vi "tableau 5 valves en liste.vi"(1 "Tableau de 5 valves":string[](array[string])=["08120001", "08120002", "08120003", "08120004", "08120005"]) -> (0 "Chaîne de 5 valves":string="08120001, 08120002, 08120003, 08120004, 08120005")   [LabVIEW 2020]
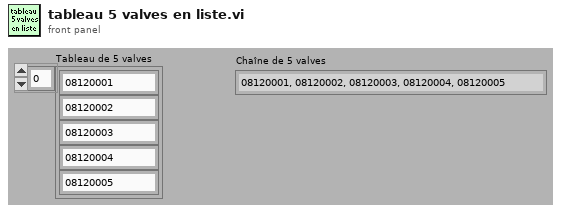
[diagram p1: front panel]
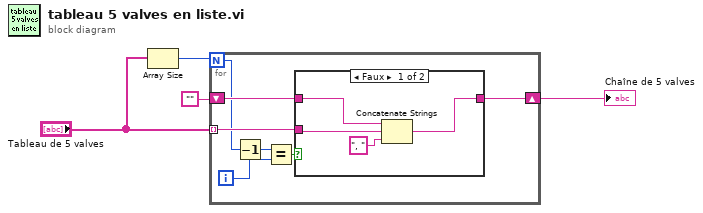
[diagram p0: block diagram]
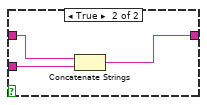
[diagram p2: hidden frame]
diagram:
  n1 = Array Size(array="Tableau de 5 valves") -> (size(s)=w3:i32)
  n2 = for {
    N: w3 -> [w7]
    tunnel: "Tableau de 5 valves" -> [w10] mode=indexing
    shift-right: [w5] -> w1
    shift-left: "" -> [w11]
    i -> [w8]
    n3 = Decrement(x=w7) -> (x-1=w6:i32)
    n4 = Equal?(x=w6, y=w8) -> (x = y?=w9:bool)
    n5 = case shown="Faux" w9 {
      tunnel: w11 -> [w14 w18]
      tunnel: w10 -> [w13 w17]
      tunnel: [w12 w16] -> w5
      frame False {
        n6 = Concatenate Strings(w14, w13, ", ") -> (w12:string)
      }
      frame True {
        n7 = Concatenate Strings(w18, w17) -> (w16:string)
      }
    }
  }
  "Chaîne de 5 valves" <- w1
